vi "Wait for Next Command.vi"(0 "VISA resource name":refnum<visa-resource-name>, 11 "error in (no error)":errorcluster) -> (4 "VISA resource name out":refnum<visa-resource-name>, 15 "error out":errorcluster)   [LabVIEW 2014, in "Associated Power Technologies 8500 Series.lvlib"]
doc: "Set the Wait to Continue flag to prevent the instrument from executing any further query or commands until the no-operation-pending flag is set to True."
uses:
  <instrlib>/Associated Power Technologies 8500 Series/Associated Power Technologies 8500 Series.lvlib
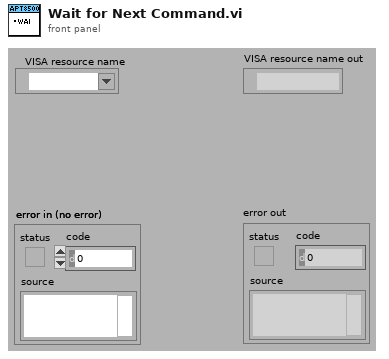
[diagram p1: front panel]
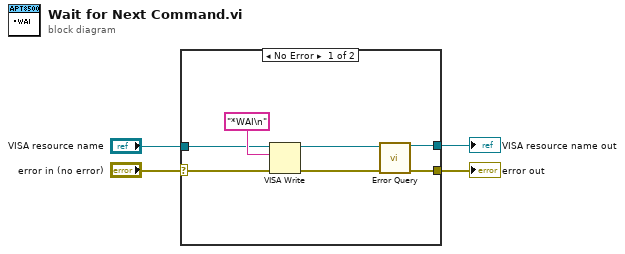
[diagram p0: block diagram]
diagram:
  n1 = case shown="No Error" "error in (no error)" {
    selector: "error in (no error)" -> [w7 w12]
    tunnel: "VISA resource name" -> [w10 w13]
    tunnel: [w9 w13] -> w3
    tunnel: [w8 w12] -> w2
    frame No Error {
      n2 = VISA Write(VISA resource name=w10, write buffer="*WAI\n" ("Command to Send (empty)"), error in (no error)=w7) -> (VISA resource name out=w6:refnum<visa-resource-name>, error out=w5:errorcluster)  [unwired: 1 out]
      n3 = call <instrlib>:"Error Query.vi"("VISA resource name"=w6, "error in (no error)"=w5) -> ("VISA resource name out"=w9:refnum<visa-resource-name>, "error out"=w8:errorcluster)  [unwired: 10 in, 2 out]
    }
    frame Error {
    }
  }
  "error out" <- w2
  "VISA resource name out" <- w3
